vi "Finish.vi"(8 "error in (no error)":errorcluster) -> ()   [LabVIEW 2013, in "VirtualRobot.lvlib"]
uses:
  VirtualRobot.lvlib
  <vilib>/ActorFramework/Message Enqueuer/Message Enqueuer.lvclass/Message Enqueuer.ctl
  <vilib>/ActorFramework/Message Enqueuer/Enqueue.vi
  Global Variables.vi
  <vilib>/ActorFramework/Message Priority Queue/Priority Enqueue.vi
  <vilib>/ActorFramework/Stop Msg/Stop Msg.lvclass
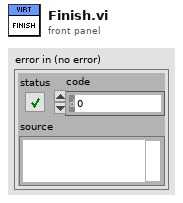
[diagram p1: front panel]
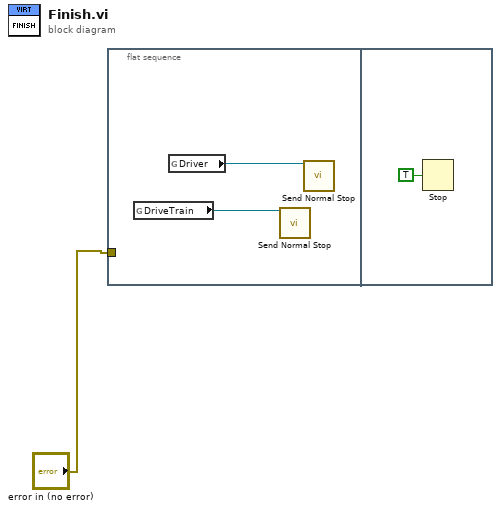
[diagram p0: block diagram]
diagram:
  n1 = flat-sequence {
    tunnel: "error in (no error)" -> [_]
    frame #0 {
      n2 = global read "Global Variables.vi" "DriveTrain"() -> (w2:refnum<class "Message Enqueuer.lvclass">)
      n3 = global read "Global Variables.vi" "Driver"() -> (w3:refnum<class "Message Enqueuer.lvclass">)
      n4 = call <vilib>:"Send Normal Stop.vi"("Message Enqueuer"=w2) -> ()  [unwired: 10 in, 1 out]
      n5 = call <vilib>:"Send Normal Stop.vi"("Message Enqueuer"=w3) -> ()  [unwired: 10 in, 1 out]
    }
    frame #1 {
      n6 = Stop(stop? (T)=TRUE) -> ()
    }
  }
